vi "DC Power.vi"(4 "Source Delay (Sec)":dbl, 5 "Load SMU Channel":string, 6 "Voltage Limit Range":dbl, 7 "Current Level":dbl, 8 "error in (no error)":errorcluster, 9 "Current Level Range":dbl, 10 "Voltage Limit":dbl, 11 "IVI Refnum in":refnum<k15>) -> (0 "error out":errorcluster, 1 "error out":errorcluster, 2 "current measurements":dbl[](array[numeric]), 3 "voltage measurements":dbl[](array[numeric]))   [LabVIEW 2021, in "NIDCPower T12.lvlib"]
uses:
  NIDCPower T12.lvlib
  <instrlib>/niDCPower/nidcpower.llb/niDCPower Source Mode.ctl
  <instrlib>/niDCPower/nidcpower.llb/niDCPower Wait For Event - Event.ctl
  <instrlib>/niDCPower/nidcpower.llb/niDCPower Output Function.ctl
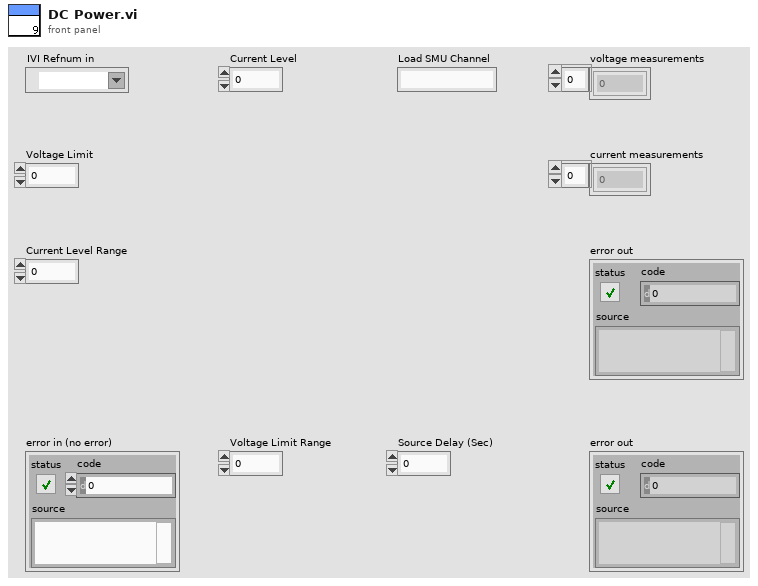
[diagram p1: front panel]
types:
  T1 = typedef "niDCPower Output Function.ctl" = i32
  T2 = typedef "niDCPower Wait For Event - Event.ctl" = i32
  T3 = typedef "niDCPower Source Mode.ctl" = i32
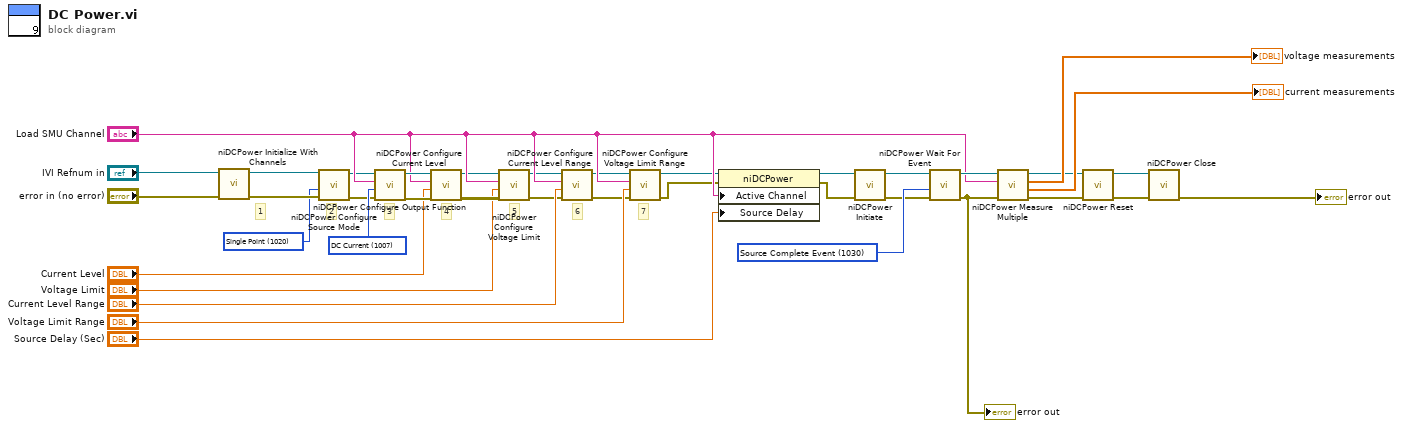
[diagram p0: block diagram]
diagram:
  w29 = T1 1007 items=["DC Voltage"=1006, "DC Current"=1007, "Pulse Voltage"=1049, "Pulse Current"=1050] ("output function")
  w26 = T2 1030 items=["Source Complete Event"=1030, "Measure Complete Event"=1031, "Sequence Iteration Complete Event"=1032, "Sequence Engine Done Event"=1033] ("event")
  w7 = T3 1020 items=["Single Point"=1020, "Sequence"=1021] ("source mode")
  # "7"
  # "6"
  # "2"
  # "3"
  # "5"
  # "4"
  # "1"
  n1 = call <instrlib>:"niDCPower Initialize With Channels.vi"("error in (no error)"="error in (no error)", "resource name"="IVI Refnum in") -> ("error out"=w35:errorcluster, "instrument handle out"=w33:refnum<k15>)  [unwired: 8 in]
  n2 = call <instrlib>:"niDCPower Configure Source Mode.vi"("error in (no error)"=w35, "source mode"=w7, "instrument handle"=w33) -> ("error out"=w5:errorcluster, "instrument handle out"=w6:refnum<k15>)  [unwired: 7 out]
  n3 = call <instrlib>:"niDCPower Configure Output Function.vi"("error in (no error)"=w5, "output function"=w29, "channel name"="Load SMU Channel", "instrument handle"=w6) -> ("error out"=w27:errorcluster, "instrument handle out"=w28:refnum<k15>)  [unwired: 6 out]
  n4 = call <instrlib>:"niDCPower Configure Current Level.vi"("error in (no error)"=w27, "current level"="Current Level", "channel name"="Load SMU Channel", "instrument handle"=w28) -> ("error out"=w2:errorcluster, "instrument handle out"=w1:refnum<k15>)  [unwired: 6 out]
  n5 = call <instrlib>:"niDCPower Configure Voltage Limit.vi"("error in (no error)"=w2, "voltage limit"="Voltage Limit", "channel name"="Load SMU Channel", "instrument handle"=w1) -> ("error out"=w8:errorcluster, "instrument handle out"=w9:refnum<k15>)  [unwired: 6 out]
  n6 = call <instrlib>:"niDCPower Configure Current Level Range.vi"("error in (no error)"=w8, "current level range"="Current Level Range", "channel name"="Load SMU Channel", "instrument handle"=w9) -> ("error out"=w10:errorcluster, "instrument handle out"=w11:refnum<k15>)  [unwired: 6 out]
  n7 = call <instrlib>:"niDCPower Configure Voltage Limit Range.vi"("error in (no error)"=w10, "voltage limit range"="Voltage Limit Range", "channel name"="Load SMU Channel", "instrument handle"=w11) -> ("error out"=w18:errorcluster, "instrument handle out"=w17:refnum<k15>)  [unwired: 6 out]
  n8 = property class="niDCPower"(reference=w17, error in=w18, "Active Channel"="Load SMU Channel", "Source Delay"="Source Delay (Sec)") -> (reference out=w20:refnum<k15>, error out=w19:errorcluster)
  n9 = call <instrlib>:"niDCPower Initiate.vi"("error in (no error)"=w19, "instrument handle"=w20) -> ("error out"=w25:errorcluster, "instrument handle out"=w23:refnum<k15>)  [unwired: 2 in, 6 out]
  n10 = call <instrlib>:"niDCPower Wait For Event.vi"("error in (no error)"=w25, "event"=w26, "instrument handle"=w23) -> ("error out"=w36:errorcluster, "instrument handle out"=w24:refnum<k15>)  [unwired: 1 in, 6 out]
  "error out" <- w36
  n11 = call <instrlib>:"niDCPower Measure Multiple.vi"("error in (no error)"=w36, "channel name"="Load SMU Channel", "instrument handle"=w24) -> ("error out"=w31:errorcluster, "current measurements"=→"current measurements":dbl[], "voltage measurements"=→"voltage measurements":dbl[], "instrument handle out"=w14:refnum<k15>)  [unwired: 5 out]
  n12 = call <instrlib>:"niDCPower Reset.vi"("error in (no error)"=w31, "instrument handle"=w14) -> ("error out"=w30:errorcluster, "instrument handle out"=w38:refnum<k15>)  [unwired: 2 in, 6 out]
  n13 = call <instrlib>:"niDCPower Close.vi"("error in (no error)"=w30, "instrument handle"=w38) -> ("error out"=→"error out":errorcluster)  [unwired: 9 in]
